vi "emi_Center FP in FP.vi"(5 "VI To position Refnum(This vi)":refnum<vi>, 7 "VI Anchor Refnum(Caller)":refnum<vi>, 9 "error in (no error)":errorcluster) -> (6 "VI to Position Refnum":refnum<vi>, 8 "VI Anchor Refnum":refnum<vi>, 10 "error out":errorcluster)   [LabVIEW 2011]
doc: "Positions \"Vi to Position\" relative to \"Vi Anchor\"\n\nIf no VI ref in, then the VI containing this VI is used.\nIf VI has multiple panes, only the first pane will be used.\n\nOn error in: Does not run."
uses:
  <vilib>/Utility/miscctls.llb/LVRectTypeDef.ctl
panel:
  # "V center>>"
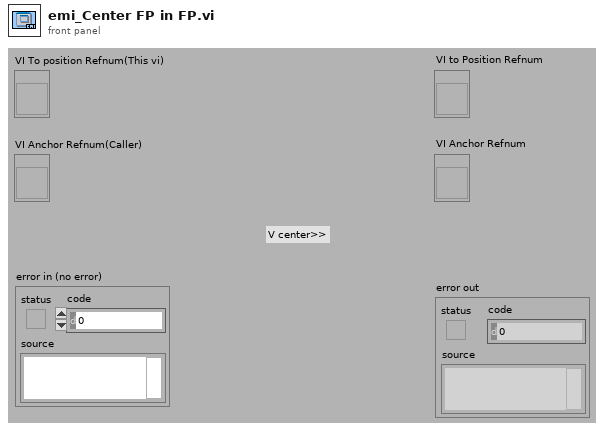
[diagram p1: front panel]
types:
  T1 = typedef "LVRectTypeDef.ctl" = cluster{"Left":i16, "Top":i16, "Right":i16, "Bottom":i16}
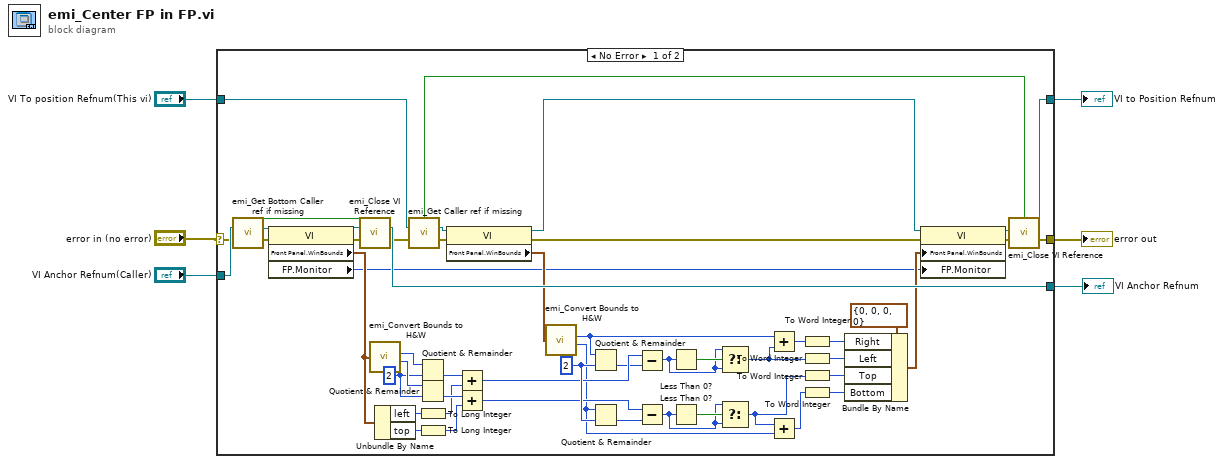
[diagram p0: block diagram]
diagram:
  n1 = case shown="No Error" "error in (no error)" {
    selector: "error in (no error)" -> [w47 w61]
    tunnel: [w44 w61] -> w6
    tunnel: "VI To position Refnum(This vi)" -> [w57 w60]
    tunnel: [w54 w60] -> w4
    tunnel: "VI Anchor Refnum(Caller)" -> [w48 w59]
    tunnel: [w46 w59] -> w1
    frame No Error {
      w35 = 2 ("y")
      w36 = 2 ("y")
      n2 = call "emi_Get Bottom Caller ref if missing.vi"("VI Refnum(Calling VI)"=w48, "error in (no error)"=w47) -> ("Ref Generated"=w51:bool, "VI Refnum Out"=w50:refnum<vi>, "error out"=w53:errorcluster)  [unwired: 11 in]
      n3 = property class="VI"(reference=w50, error in=w53) -> (reference out=w49:refnum<vi>, error out=w52:errorcluster, "Front Panel.WinBounds"=w39:T1, "FP.Monitor"=w9:u16)
      n4 = call "emi_Close VI Reference.vi"("Close ref?(T)"=w51, "VI Refnum"=w49, "error in (no error)"=w52) -> ("VI Refnum Out"=w46:refnum<vi>, "error out"=w45:errorcluster)  [unwired: 11 in]
      n5 = call "emi_Convert Bounds to H&W.vi"("Bounds"=w39) -> ("Width"=w38:i32, "Height"=w37:i32)  [unwired: 6 in]
      n6 = Unbundle By Name(w39) -> ("left"=w29:i16, "top"=w32:i16)
      n7 = call "emi_Get Caller ref if missing.vi"("VI Refnum(Calling VI)"=w57, "error in (no error)"=w45) -> ("Ref Generated"=w58:bool, "VI Refnum Out"=w55:refnum<vi>, "error out"=w56:errorcluster)  [unwired: 11 in]
      n8 = Quotient & Remainder(x=w38, y=w36) -> (floor(x/y)=w30:i32)  [unwired: 1 out]
      n9 = Quotient & Remainder(x=w37, y=w36) -> (floor(x/y)=w33:i32)  [unwired: 1 out]
      n10 = To Long Integer(number=w29) -> (32bit integer=w28:i32)
      n11 = To Long Integer(number=w32) -> (32bit integer=w31:i32)
      n12 = property class="VI"(reference=w55, error in=w56) -> (reference out=w41:refnum<vi>, error out=w42:errorcluster, "Front Panel.WinBounds"=w34:T1)
      n13 = Add(x=w30, y=w28) -> (x+y=w27:i32)
      n14 = Add(x=w33, y=w31) -> (x+y=w25:i32)
      n15 = call "emi_Convert Bounds to H&W.vi"("Bounds"=w34) -> ("Width"=w21:i32, "Height"=w18:i32)  [unwired: 6 in]
      n16 = Quotient & Remainder(x=w21, y=w35) -> (floor(x/y)=w26:i32)  [unwired: 1 out]
      n17 = Quotient & Remainder(x=w18, y=w35) -> (floor(x/y)=w24:i32)  [unwired: 1 out]
      n18 = Subtract(x=w27, y=w26) -> (x-y=w8:i32)
      n19 = Subtract(x=w25, y=w24) -> (x-y=w7:i32)
      n20 = Less Than 0?(x=w8) -> (x < 0?=w13:bool)
      n21 = Less Than 0?(x=w7) -> (x < 0?=w11:bool)
      n22 = Select(t=w8, s=w13, f=w8) -> (s? t:f=w12:i32)
      n23 = Select(t=w7, s=w11, f=w7) -> (s? t:f=w10:i32)
      n24 = Add(x=w21, y=w12) -> (x+y=w20:i32)
      n25 = Add(x=w10, y=w18) -> (x+y=w19:i32)
      n26 = To Word Integer(number=w20) -> (16bit integer=w17:i16)
      n27 = To Word Integer(number=w12) -> (16bit integer=w16:i16)
      n28 = To Word Integer(number=w10) -> (16bit integer=w15:i16)
      n29 = To Word Integer(number=w19) -> (16bit integer=w14:i16)
      n30 = Bundle By Name(cluster=T1 {"Left"=0, "Top"=0, "Right"=0, "Bottom"=0} ("Front Panel Window:Window Bounds"), "Right"=w17, "Left"=w16, "Top"=w15, "Bottom"=w14) -> (w23:T1)
      n31 = property class="VI"(reference=w41, error in=w42, "Front Panel.WinBounds"=w23, "FP.Monitor"=w9) -> (reference out=w40:refnum<vi>, error out=w43:errorcluster)
      n32 = call "emi_Close VI Reference.vi"("Close ref?(T)"=w58, "VI Refnum"=w40, "error in (no error)"=w43) -> ("VI Refnum Out"=w54:refnum<vi>, "error out"=w44:errorcluster)  [unwired: 11 in]
    }
    frame Error {
    }
  }
  "error out" <- w6
  "VI to Position Refnum" <- w4
  "VI Anchor Refnum" <- w1
